vi "SelectValidRobot.vi"(0 "Utilities in":refnum<class "Utilities.lvclass">, 5 "Robot 1":refnum<class "Robot.lvclass">, 7 "Robot 2":refnum<class "Robot.lvclass">, 9 "Robot 3":refnum<class "Robot.lvclass">, 11 "error in (no error)":errorcluster) -> (4 "Utilities out":refnum<class "Utilities.lvclass">, 6 "Robot out":refnum<class "Robot.lvclass">, 15 "error out":errorcluster)   [LabVIEW 2018, in "Utilities.lvclass"]
uses:
  Utilities.lvclass
  Robot_class/Robot.lvclass
  Robot_class/Robot.lvclass/Robot.ctl
  Robot_class/Read id.vi
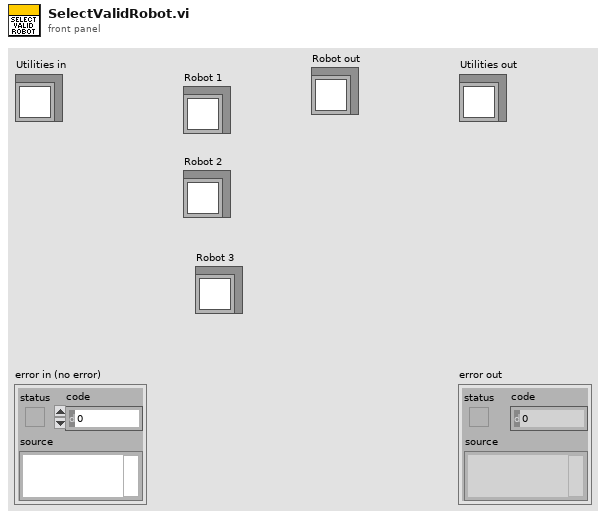
[diagram p1: front panel]
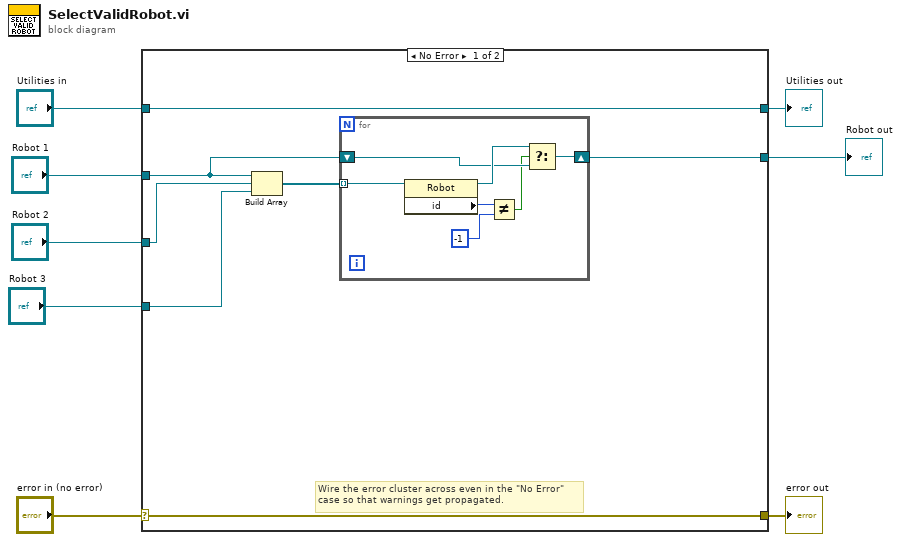
[diagram p0: block diagram]
diagram:
  n1 = case shown="No Error" "error in (no error)" {
    selector: "error in (no error)" -> [w14 w25]
    tunnel: [w14 w25] -> w7
    tunnel: [w15 w24] -> w5
    tunnel: "Utilities in" -> [w15 w24]
    tunnel: "Robot 1" -> [w9 w23]
    tunnel: "Robot 2" -> [w13 _]
    tunnel: "Robot 3" -> [w12 _]
    tunnel: [w10 w23] -> w1
    frame No Error {
      # "Wire the error cluster across even in the \"No Error\"\ncase so that warnings get propagated."
      n2 = Build Array(w9, w13, w12) -> (w11:refnum<class "Robot.lvclass">[])
      n3 = for {
        tunnel: w11 -> [w22] mode=indexing
        shift-right: [w21] -> w10
        shift-left: w9 -> [w19]
        n4 = property class="Robot"(reference=w22) -> (reference out=w20:refnum<class "Robot.lvclass">, "id"=w18:i32)  [unwired: 1 in, 1 out]
        n5 = Not Equal?(x=w18, y=-1) -> (x != y?=w16:bool)
        n6 = Select(t=w20, s=w16, f=w19) -> (s? t:f=w21:refnum<class "Robot.lvclass">)
      }
    }
    frame Error {
    }
  }
  "error out" <- w7
  "Utilities out" <- w5
  "Robot out" <- w1
